vi "Acquire data -- subVI.vi"(7 "N samples":i32=1 caption="Muestras", 8 "error in (no error)":errorcluster, 9 "Average":bool, 11 "Data Cluster":T2 {"Interval" format="%#_gnm"; "Current position" format="%#_gnm"}) -> (0 "error out":errorcluster, 1 "event data":T1, 2 "Measurement":dbl, 3 "Data Cluster":T2 {"Interval" format="%#_gnm"; "Current position" format="%#_gnm"})   [LabVIEW 2020]
uses:
  controls/UI Data.ctl
  controls/Lock-in config.ctl
  controls/Mono config.ctl
  controls/Wake HL data -- cluster.ctl
  Lock-in-amplifier/Libraries/Lock-in amplifier/Lock-in amplifier.lvlib
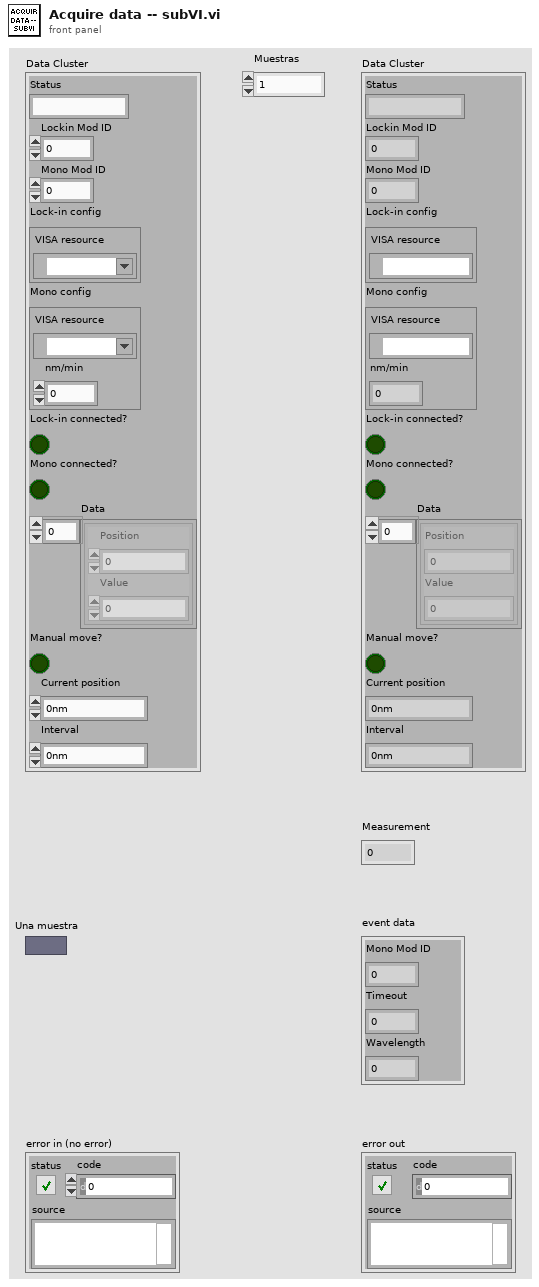
[diagram p1: front panel]
types:
  T1 = typedef "Wake HL data -- cluster.ctl" = cluster{"Mono Mod ID":i32, "Timeout":i32, "Wavelength":dbl}
  T2 = typedef "UI Data.ctl" = cluster{"Status":string, "Lockin Mod ID":i32, "Mono Mod ID":i32, "Lock-in config":T3, "Mono config":T4, "Lock-in connected?":bool, "Mono connected?":bool, "Data":cluster{"Position":dbl, "Value":dbl}[], "Manual move?":bool, "Current position":dbl, "Interval":dbl}
  T3 = typedef "Lock-in config.ctl" = cluster{"VISA resource ":refnum<visa-resource-name>}
  T4 = typedef "Mono config.ctl" = cluster{"VISA resource ":refnum<visa-resource-name>, "nm/min":dbl}
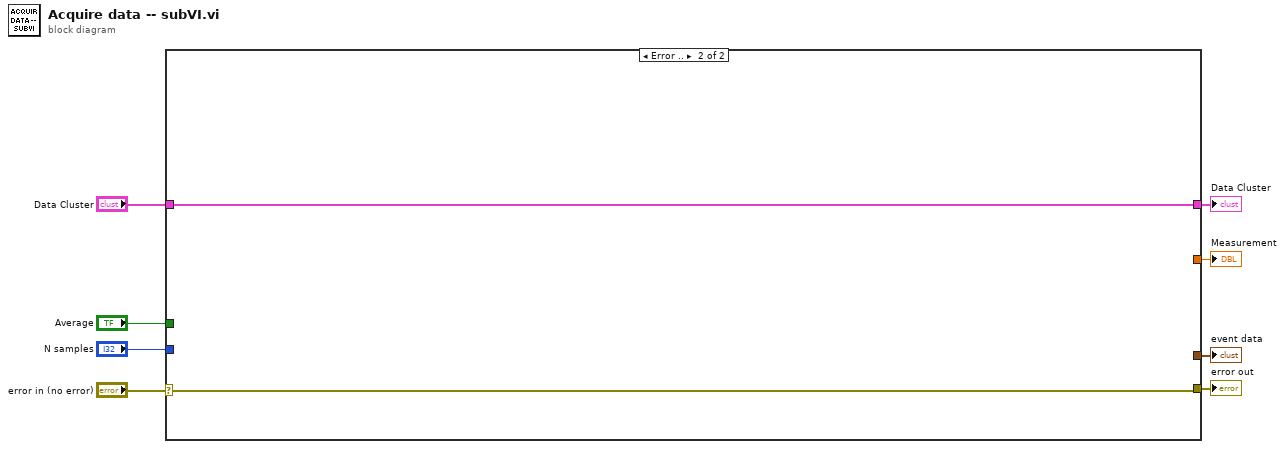
[diagram p0: block diagram]
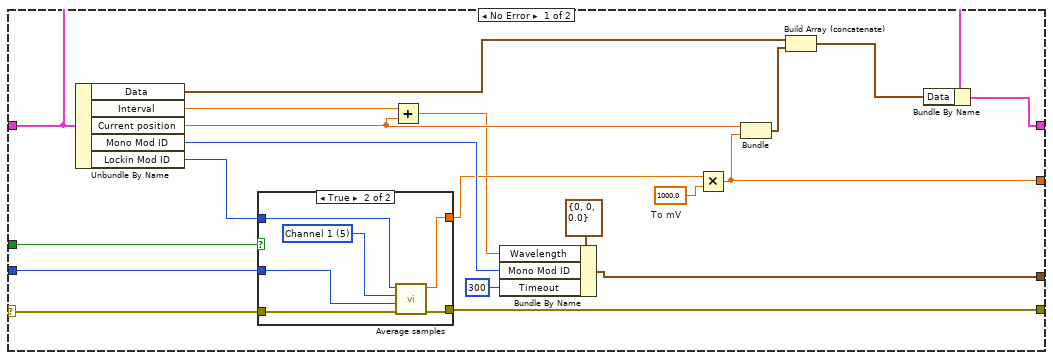
[diagram p2: hidden frame]
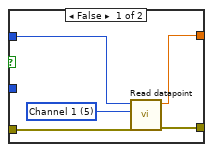
[diagram p3: hidden frame]
diagram:
  n1 = case shown="Error .." "error in (no error)" {
    selector: "error in (no error)" -> [w19 w40]
    tunnel: [w23 w40] -> w8
    tunnel: [w21 _] -> w7
    tunnel: "Average" -> [w18 _]
    tunnel: "N samples" -> [w16 _]
    tunnel: "Data Cluster" -> [w13 w41]
    tunnel: [w12 w41] -> w2
    tunnel: [w9 _] -> w1
    frame No Error {
      w22 = 1000.0  # To mV
      n2 = Unbundle By Name(w13) -> ("Data"=w15:cluster{"Position":dbl, "Value":dbl}[], "Interval"=w27:dbl, "Current position"=w28:dbl, "Mono Mod ID"=w26:i32, "Lockin Mod ID"=w17:i32)
      n3 = case shown="True" w18 {
        tunnel: w19 -> [w33 w39]
        tunnel: [w32 w38] -> w23
        tunnel: w17 -> [w31 w37]
        tunnel: [w29 w35] -> w20
        tunnel: w16 -> [_ w34]
        frame False {
          w30 = u16 5 items=["X"=1, "Y"=2, "R"=3, "Theta"=4, "Channel 1"=5, "Channel 2"=6, "Aux In 1"=7, "Aux In 2"=8, "Aux In 3"=9, "Aux In 4"=10] ("Parameter")
          n4 = call "Read datapoint.vi"("error in"=w33, "Parameter"=w30, "Module ID"=w31) -> ("error out"=w32:errorcluster, "Data"=w29:dbl)  [unwired: 6 in, 1 out]
        }
        frame True {
          w36 = u16 5 items=["X"=1, "Y"=2, "R"=3, "Theta"=4, "Channel 1"=5, "Channel 2"=6, "Aux In 1"=7, "Aux In 2"=8, "Aux In 3"=9, "Aux In 4"=10] ("Parameter")
          n5 = call "Average samples.vi"("error in"=w39, "N samples"=w34, "Parameter"=w36, "Module ID"=w37) -> ("error out"=w38:errorcluster, "Measurement"=w35:dbl)  [unwired: 5 in, 1 out]
        }
      }
      n6 = Add(x=w27, y=w28) -> (x+y=w10:dbl)
      n7 = Bundle By Name(cluster=T1 {"Mono Mod ID"=0, "Timeout"=0, "Wavelength"=0.0} ("event data"), "Wavelength"=w10, "Mono Mod ID"=w26, "Timeout"=300) -> (w9:T1)
      n8 = Multiply(x=w20, y=w22) -> (x*y=w21:dbl)
      n9 = Bundle("Current position"=w28, w21) -> (w14:cluster{"Current position":dbl, dbl})  [unwired: 1 in]
      n10 = Build Array (concatenate)(w15, w14) -> (w11:cluster{"Current position":dbl, "Value":dbl}[])
      n11 = Bundle By Name(cluster=w13, "Data"=w11) -> (w12:T2)
    }
    frame Error {
    }
  }
  "error out" <- w8
  "Measurement" <- w7
  "Data Cluster" <- w2
  "event data" <- w1
